vi "Online_Program_redesign_For_TV_1세부.vi"() -> ()   [LabVIEW 2014]
uses:
  <vilib>/Utility/file.llb/Read From Spreadsheet File (DBL).vi
  <vilib>/Analysis/Matrix/Numeric/Conversions/Array To Matrix - RA2.vi
  <vilib>/Instr/_visa.llb/VISA Configure Serial Port (Instr).vi
  <vilib>/DAQmx/create/channels.llb/DAQmx Create Channel (AI-Voltage-Basic).vi
  <vilib>/DAQmx/configure/timing.llb/DAQmx Timing (Sample Clock).vi
  <vilib>/DAQmx/read.llb/DAQmx Read (Analog 1D Wfm NChan NSamp).vi
  <vilib>/Analysis/Matrix/Numeric/Conversions/Array To Matrix - RA.vi
  <vilib>/Utility/file.llb/Write To Spreadsheet File (DBL).vi
  <vilib>/Utility/file.llb/Write To Spreadsheet File (I64).vi
  <vilib>/Analysis/Matrix/NI_Matrix.lvlib
  NeuroSky_Dll_Call/Debug/NeuroSky_Dll_Call.dll
  user32.dll
panel:
  out "에러 출력":errorcluster
  out "메시지 2":string
  out "큐사인":bool
  out "icon_온도":bool
  out "icon_용변":bool
  out "icon_자판":bool
  out "icon_응급":bool=TRUE
  out "icon_기계":bool
  out "icon_침대":bool
  out "메시지":string
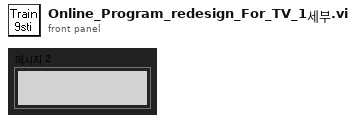
[diagram p1: front panel]
types:
  T1 = typedef "NI_Matrix.lvlib/RealMatrix.ctl" = dbl[][]
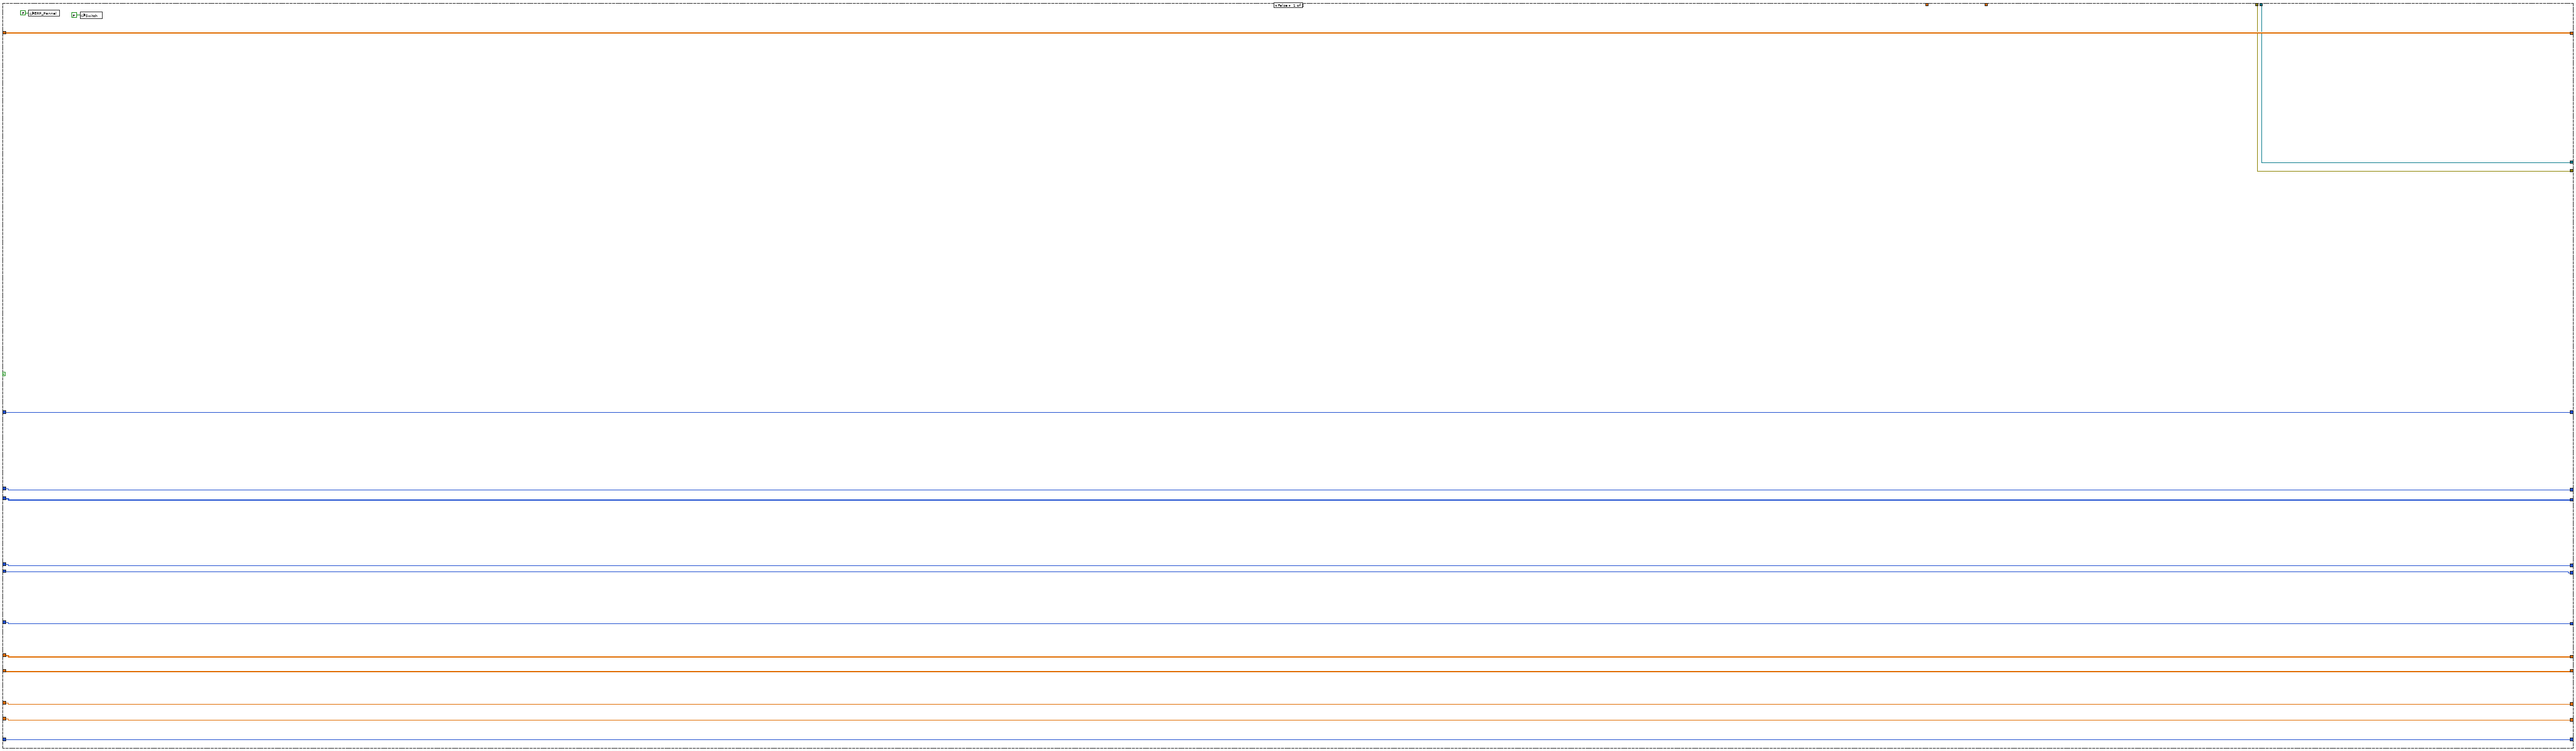
[diagram p2: hidden frame]
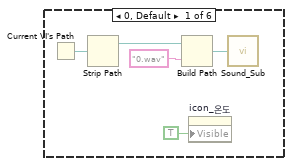
[diagram p3: hidden frame]
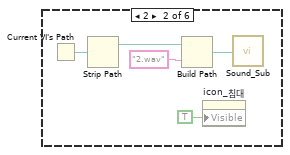
[diagram p4: hidden frame]
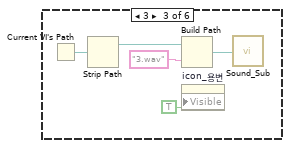
[diagram p5: hidden frame]
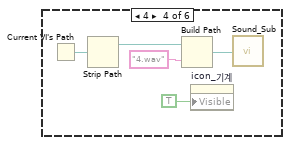
[diagram p6: hidden frame]
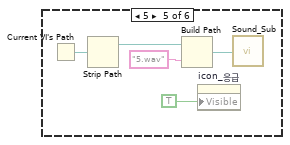
[diagram p7: hidden frame]
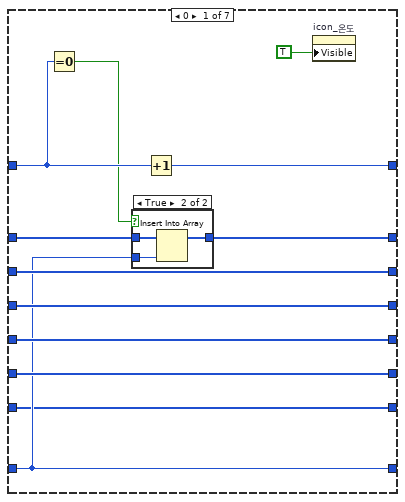
[diagram p9: hidden frame]
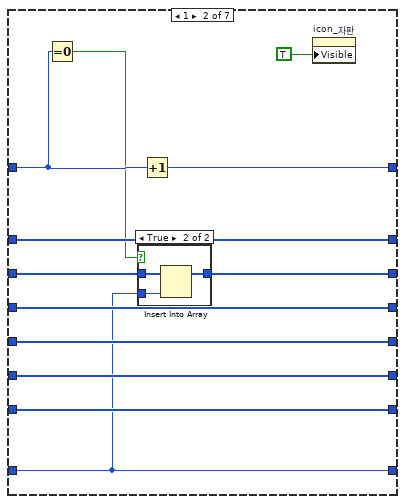
[diagram p11: hidden frame]
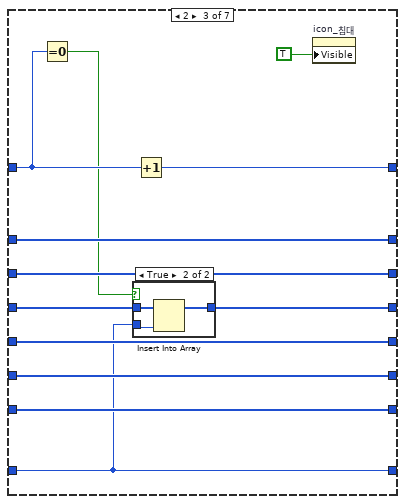
[diagram p13: hidden frame]
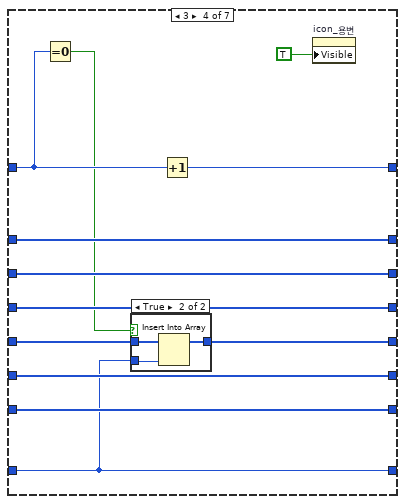
[diagram p15: hidden frame]
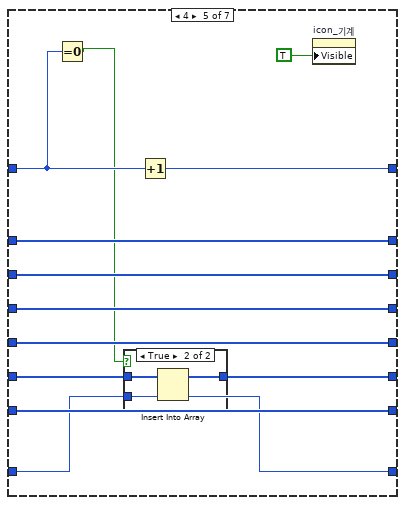
[diagram p17: hidden frame]
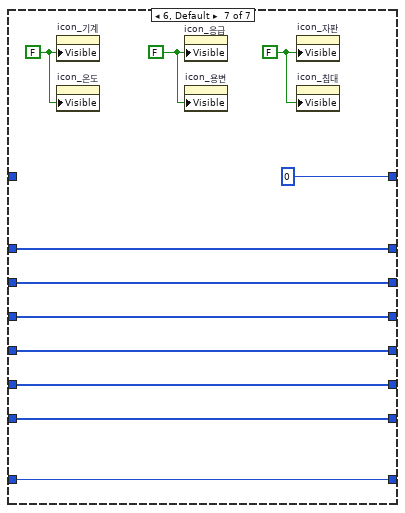
[diagram p20: hidden frame]
diagram:
  n1 = flat-sequence {
    tunnel: [w39] -> w19
    tunnel: w19 -> [w53]
    tunnel: [w53] -> w18
    tunnel: [w51] -> w17
    tunnel: [w44] -> w7
    tunnel: [w43] -> w4
    tunnel: [w40] -> w3
    tunnel: w18 -> [w72]
    tunnel: [w72] -> w16
    tunnel: [w81] -> w15
    tunnel: [w79] -> w14
    tunnel: [w77] -> w13
    tunnel: w17 -> [w61]
    tunnel: [w76] -> w12
    tunnel: [w73] -> w11
    tunnel: [w69] -> w10
    tunnel: [w67] -> w9
    tunnel: [w66] -> w8
    tunnel: w7 -> [w60]
    tunnel: [w64] -> w6
    tunnel: [w62] -> w5
    tunnel: w4 -> [w59]
    tunnel: w3 -> [w58]
    tunnel: [w57] -> w2
    tunnel: [w56] -> w1
    tunnel: w16 -> [w750]
    tunnel: w15 -> [w745]
    tunnel: w14 -> [w784]
    tunnel: w13 -> [w780]
    tunnel: w12 -> [w777]
    tunnel: w11 -> [w773]
    tunnel: w10 -> [w767]
    tunnel: w9 -> [w762]
    tunnel: w8 -> [w759]
    tunnel: w6 -> [w756]
    tunnel: w5 -> [w751]
    tunnel: w2 -> [w747]
    tunnel: w1 -> [w746]
    frame #0 {
      w20 = FALSE ("Visible")
      w22 = 500 ("Position:Left")
      # "0 = 온도\n1 = 자판\n2 = 침대\n3 = 용변 \n4 = 기계 \n5 = 응급"
      n2 = global read "Control_Panel_정리.vi" "피험자 이름"() -> (w30:string)
      n3 = Get Date/Time In Seconds() -> (seconds since 1Jan1904=w36:timestamp)
      n4 = property on="icon_기계" class="Bool (strict)"("Left"=w22, "Top"=w22) -> ()  [unwired: 2 in, 2 out]
      n5 = property on="icon_자판" class="Bool (strict)"("Left"=w22, "Top"=w22) -> ()  [unwired: 2 in, 2 out]
      n6 = property on="icon_침대" class="Bool (strict)"("Left"=w22, "Top"=w22) -> ()  [unwired: 2 in, 2 out]
      n7 = property on="icon_온도" class="Bool (strict)"("Left"=w22, "Top"=w22) -> ()  [unwired: 2 in, 2 out]
      n8 = property on="icon_용변" class="Bool (strict)"("Left"=w22, "Top"=w22) -> ()  [unwired: 2 in, 2 out]
      n9 = property on="icon_응급" class="Bool (strict)"("Left"=w22, "Top"=w22) -> ()  [unwired: 2 in, 2 out]
      n10 = property on="큐사인" class="Bool (strict)"("Left"=w22, "Top"=w22) -> ()  [unwired: 2 in, 2 out]
      n11 = Get Date/Time String(seconds (now)=w36) -> (date string=w37:string)  [unwired: 2 in, 1 out]
      n12 = Concatenate Strings("Emotion_Research\\" ("string"), w30, "_Online(Step2)\\" ("문자열")) -> (w32:string)
      n13 = Concatenate Strings(w32, w37) -> (w34:string)
      n14 = Build Path(base path=path "C:/" ("path"), name or relative path=w34) -> (appended path=w35:path)
      n15 = property on="icon_기계" class="Bool (strict)"("Visible"=w20) -> ()  [unwired: 2 in, 2 out]
      n16 = property on="icon_온도" class="Bool (strict)"("Visible"=w20) -> ()  [unwired: 2 in, 2 out]
      n17 = property on="icon_용변" class="Bool (strict)"("Visible"=w20) -> ()  [unwired: 2 in, 2 out]
      n18 = property on="icon_응급" class="Bool (strict)"("Visible"=w20) -> ()  [unwired: 2 in, 2 out]
      n19 = property on="icon_자판" class="Bool (strict)"("Visible"=w20) -> ()  [unwired: 2 in, 2 out]
      n20 = property on="icon_침대" class="Bool (strict)"("Visible"=w20) -> ()  [unwired: 2 in, 2 out]
      n21 = property on="큐사인" class="Bool (strict)"("Visible"=w20) -> ()  [unwired: 2 in, 2 out]
      n22 = Create Folder(path (use dialog)=w35) -> (created path=w39:path, error out=→"에러 출력":errorcluster)  [unwired: 2 in, 1 out]
      "icon_온도" <- FALSE ("icon_전원 6")
      "icon_용변" <- FALSE ("icon_전체종료")
      "icon_자판" <- FALSE ("icon_음량업 2")
      "icon_응급" <- FALSE ("icon_채널다운")
      "icon_기계" <- FALSE ("icon_음량다")
      "icon_침대" <- FALSE ("icon_채널업")
      "큐사인" <- FALSE ("icon_전원 7")
    }
    frame #1 {
      w47 = 1 ("인덱스 (행)")
      # "call SWLDA in matrix"
      # "call SWLDA LDA matrix"
      # "Device Control Part\ncall dll to communicate with\nNeuroSky MindWave System"
      n23 = while {
        stop <- w54 stop-if-true
        n24 = global read "Control_Panel_정리.vi" "Start"() -> (w54:bool)
      }
      n25 = global read "Control_Panel_정리.vi" "VISA resource name"() -> (w41:refnum<visa-resource-name>)
      n26 = global read "Control_Panel_정리.vi" "in"() -> (w45:path)
      n27 = global read "Control_Panel_정리.vi" "LDA_Matrix"() -> (w50:path)
      n28 = call-poly "VISA Configure Serial Port"("VISA resource name"=w41, "baud rate (9600)"=u32 115200) -> ("VISA resource name out"=w43:refnum<visa-resource-name>, "error out"=w40:errorcluster)  [unwired: 12 in]
      n29 = call-poly <vilib>:"Read From Spreadsheet File.vi"("format (%.3f)"="%.6f", "file path (dialog if empty)"=w45) -> ("all rows"=w46:dbl[][])  [unwired: 5 in, 4 out]
      n30 = call-poly <vilib>:"Read From Spreadsheet File.vi"("format (%.3f)"="%.6f", "file path (dialog if empty)"=w50) -> ("all rows"=w51:dbl[][])  [unwired: 5 in, 4 out]
      n31 = global write "Control_Panel_정리.vi" "error out"(w40) -> ()
      n32 = Delete From Array(array=w46, length=w47, index (row)=w47) -> (array with subset deleted=w48:dbl[][])  [unwired: 1 in, 1 out]
      n33 = call-poly <vilib>:"Array To Matrix.vi"("Real 2D Array"=w48) -> ("Real Matrix"=w44:T1)
    }
    frame #2 {
      w65 = dbl[] []
      w63 = dbl[][] []
      w68 = i16[] []
      n34 = while {
        shift-right: [w89] -> w81
        shift-left: dbl[][] [] -> [w95]
        shift-right: [w115] -> _
        shift-left: 0 ("y") -> [w116]
        shift-right: [w109] -> w79
        shift-left: i32[][] [] -> [w110]
        shift-right: [w113] -> w77
        shift-left: i32[] [] -> [w114]
        shift-right: [w111] -> w76
        shift-left: w68 -> [w112]
        shift-right: [w107] -> w73
        shift-left: w68 -> [w108]
        shift-right: [w106] -> w69
        shift-left: w68 -> [w105]
        shift-right: [w104] -> w67
        shift-left: w63 -> [w103]
        shift-right: [w102] -> w66
        shift-left: w65 -> [w101]
        shift-right: [w100] -> w64
        shift-left: w65 -> [w99]
        shift-right: [w98] -> w62
        shift-left: w63 -> [w97]
        tunnel: w61 -> [w96]
        tunnel: w60 -> [w94]
        tunnel: [w92] -> _
        tunnel: w59 -> [w92]
        tunnel: w58 -> [w93]
        tunnel: [w91] -> w57
        tunnel: [w90] -> w56
        shift-right: [w83] -> _
        shift-left: 0 -> [w84]
        stop <- w85 stop-if-true
        n35 = global read "Control_Panel_정리.vi" "Receive_Interaction"() -> (w87:u8)
        n36 = global read "Control_Panel_정리.vi" "Switch"() -> (w86:bool)
        n37 = dll-call lib="User32.dll" fn="GetAsyncKeyState"("vKey"=w87) -> ("return type"=w88:i64)  [unwired: 4 in, 2 out]
        n38 = Not Equal To 0?(x=w88) -> (x != 0?=w82:bool)
        n39 = Or(x=w82, y=w86) -> ()  [unwired: 1 out]
        n40 = case shown="True" w82 {
          tunnel: w116 -> [w127 w164]
          tunnel: [w127 w163] -> w115
          tunnel: w114 -> [w126 w162]
          tunnel: [w126 w161] -> w113
          tunnel: w112 -> [w123 w160]
          tunnel: [w123 w159] -> w111
          tunnel: w110 -> [w125 w158]
          tunnel: [w125 w157] -> w109
          tunnel: w108 -> [w124 w156]
          tunnel: [w124 w155] -> w107
          tunnel: [w122 w154] -> w106
          tunnel: w105 -> [w122 w153]
          tunnel: [w121 w152] -> w104
          tunnel: w103 -> [w121 w151]
          tunnel: [w119 w150] -> w102
          tunnel: w101 -> [w119 w149]
          tunnel: [w118 w148] -> w100
          tunnel: w99 -> [w118 w147]
          tunnel: [w120 w146] -> w98
          tunnel: w97 -> [w120 w145]
          tunnel: w96 -> [_ w144]
          tunnel: w95 -> [w130 w143]
          tunnel: w94 -> [_ w141]
          tunnel: w93 -> [w128 w140]
          tunnel: w92 -> [w129 w139]
          tunnel: [w129 w138] -> w91
          tunnel: [w128 w137] -> w90
          tunnel: [w130 w136] -> w89
          tunnel: w84 -> [w117 w134]
          tunnel: [w117 w133] -> w83
          frame False {
            n41 = global write "Control_Panel_정리.vi" "ERP_Pannel"(FALSE ("ERP_Pannel")) -> ()
            n42 = global write "Control_Panel_정리.vi" "Switch"(FALSE ("Switch")) -> ()
          }
          frame True {
            n43 = global write "Control_Panel_정리.vi" "ERP_Pannel"(TRUE ("ERP_Pannel")) -> ()
            n44 = flat-sequence {
              tunnel: [w216] -> w202
              tunnel: w164 -> [w215]
              tunnel: [w215] -> w201
              tunnel: [w203] -> w200
              tunnel: w162 -> [w212]
              tunnel: [w212] -> w199
              tunnel: w160 -> [w211]
              tunnel: [w211] -> w198
              tunnel: w158 -> [w210]
              tunnel: [w210] -> w197
              tunnel: [w209] -> w196
              tunnel: w156 -> [w209]
              tunnel: w153 -> [w208]
              tunnel: [w208] -> w195
              tunnel: w151 -> [w207]
              tunnel: [w207] -> w194
              tunnel: w149 -> [w206]
              tunnel: [w206] -> w193
              tunnel: w147 -> [w205]
              tunnel: [w205] -> w192
              tunnel: w145 -> [w204]
              tunnel: [w204] -> w191
              tunnel: w202 -> [w278]
              tunnel: w201 -> [w275]
              tunnel: [w276] -> w190
              tunnel: [w265] -> w189
              tunnel: [w274] -> w188
              tunnel: [w273] -> w187
              tunnel: w200 -> [w272]
              tunnel: [w272] -> w186
              tunnel: w199 -> [w271]
              tunnel: [w271] -> w185
              tunnel: [w270] -> w184
              tunnel: w198 -> [w270]
              tunnel: [w269] -> w183
              tunnel: w197 -> [w269]
              tunnel: [w268] -> w182
              tunnel: w196 -> [w268]
              tunnel: [w267] -> w181
              tunnel: w195 -> [w267]
              tunnel: [w266] -> w180
              tunnel: w194 -> [w266]
              tunnel: [w264] -> w179
              tunnel: w193 -> [w264]
              tunnel: [w263] -> w178
              tunnel: w192 -> [w263]
              tunnel: w191 -> [w262]
              tunnel: [w262] -> w177
              tunnel: w190 -> [w508]
              tunnel: w189 -> [w480]
              tunnel: w188 -> [w521]
              tunnel: w187 -> [w522]
              tunnel: w134 -> [w520]
              tunnel: [w521] -> w166
              tunnel: [w481] -> w167
              tunnel: w186 -> [w507]
              tunnel: w185 -> [w516]
              tunnel: [w515] -> w168
              tunnel: w184 -> [w513]
              tunnel: [w512] -> w169
              tunnel: w183 -> [w511]
              tunnel: [w509] -> w170
              tunnel: w182 -> [w506]
              tunnel: [w505] -> w171
              tunnel: [w503] -> w172
              tunnel: w181 -> [w502]
              tunnel: [w500] -> w173
              tunnel: w180 -> [w499]
              tunnel: [w497] -> w174
              tunnel: w179 -> [w496]
              tunnel: [w494] -> w175
              tunnel: w178 -> [w493]
              tunnel: [w490] -> w176
              tunnel: w177 -> [w489]
              tunnel: w144 -> [w488]
              tunnel: [w480] -> w142
              tunnel: w141 -> [w484]
              tunnel: [w483] -> w165
              tunnel: [w543] -> w163
              tunnel: [w542] -> w161
              tunnel: [w539] -> w159
              tunnel: [w541] -> w157
              tunnel: [w540] -> w155
              tunnel: [w538] -> w154
              tunnel: [w537] -> w152
              tunnel: [w536] -> w150
              tunnel: [w535] -> w148
              tunnel: [w534] -> w146
              tunnel: w176 -> [w534]
              tunnel: w175 -> [w535]
              tunnel: w174 -> [w536]
              tunnel: w173 -> [w537]
              tunnel: w172 -> [w538]
              tunnel: w171 -> [w540]
              tunnel: w170 -> [w541]
              tunnel: w169 -> [w539]
              tunnel: w168 -> [w542]
              tunnel: w167 -> [w533]
              tunnel: w166 -> [w543]
              tunnel: w165 -> [w532]
              tunnel: w140 -> [w531]
              tunnel: w139 -> [w530]
              tunnel: [w529] -> w138
              tunnel: [w528] -> w137
              frame #0 {
                # "결과로 만들어지는 배열은 일차원배열로\n출력되면 랜덤 숫자는 0부터 시작함"
                n45 = global read "Control_Panel_정리.vi" "Target_Command"() -> (w203:i32)
                n46 = global read "Control_Panel_정리.vi" "Flash_Repeat"() -> (w214:i32)
                n47 = global read "Control_Panel_정리.vi" "Random_num"() -> (w213:i32)
                n48 = disable-structure shown="비활성화" {
                  disable-tunnel: w203 -> [w217 _]
                  frame Disabled {
                    n49 = case shown="1" w217 {
                      frame 0, Default {
                        n50 = Current VI's Path() -> (path=w220:path)
                        n51 = Strip Path(path=w220) -> (stripped path=w221:path)  [unwired: 1 out]
                        n52 = Build Path(base path=w221, name or relative path="0.wav" ("이름 또는 상대 경로")) -> (appended path=w219:path)
                        n53 = property on="icon_온도" class="Bool (strict)"("Visible"=TRUE) -> ()  [unwired: 2 in, 2 out]
                        n54 = call "Sound_Sub.vi"("path"=w219) -> ()
                      }
                      frame 2 {
                        n55 = Current VI's Path() -> (path=w224:path)
                        n56 = Strip Path(path=w224) -> (stripped path=w225:path)  [unwired: 1 out]
                        n57 = Build Path(base path=w225, name or relative path="2.wav" ("이름 또는 상대 경로")) -> (appended path=w227:path)
                        n58 = property on="icon_침대" class="Bool (strict)"("Visible"=TRUE) -> ()  [unwired: 2 in, 2 out]
                        n59 = call "Sound_Sub.vi"("path"=w227) -> ()
                      }
                      frame 3 {
                        n60 = Current VI's Path() -> (path=w229:path)
                        n61 = Strip Path(path=w229) -> (stripped path=w230:path)  [unwired: 1 out]
                        n62 = Build Path(base path=w230, name or relative path="3.wav" ("이름 또는 상대 경로")) -> (appended path=w232:path)
                        n63 = property on="icon_용변" class="Bool (strict)"("Visible"=TRUE) -> ()  [unwired: 2 in, 2 out]
                        n64 = call "Sound_Sub.vi"("path"=w232) -> ()
                      }
                      frame 4 {
                        n65 = Current VI's Path() -> (path=w234:path)
                        n66 = Strip Path(path=w234) -> (stripped path=w235:path)  [unwired: 1 out]
                        n67 = Build Path(base path=w235, name or relative path="4.wav" ("이름 또는 상대 경로")) -> (appended path=w237:path)
                        n68 = property on="icon_기계" class="Bool (strict)"("Visible"=TRUE) -> ()  [unwired: 2 in, 2 out]
                        n69 = call "Sound_Sub.vi"("path"=w237) -> ()
                      }
                      frame 5 {
                        n70 = Current VI's Path() -> (path=w239:path)
                        n71 = Strip Path(path=w239) -> (stripped path=w240:path)  [unwired: 1 out]
                        n72 = Build Path(base path=w240, name or relative path="5.wav" ("이름 또는 상대 경로")) -> (appended path=w242:path)
                        n73 = property on="icon_응급" class="Bool (strict)"("Visible"=TRUE) -> ()  [unwired: 2 in, 2 out]
                        n74 = call "Sound_Sub.vi"("path"=w242) -> ()
                      }
                      frame 1 {
                        n75 = Current VI's Path() -> (path=w245:path)
                        n76 = Strip Path(path=w245) -> (stripped path=w246:path)  [unwired: 1 out]
                        n77 = Build Path(base path=w246, name or relative path="1.wav" ("이름 또는 상대 경로")) -> (appended path=w244:path)
                        n78 = property on="icon_자판" class="Bool (strict)"("Visible"=TRUE) -> ()  [unwired: 2 in, 2 out]
                        n79 = call "Sound_Sub.vi"("path"=w244) -> ()
                      }
                    }
                  }
                  frame Enabled {
                  }
                }
                n80 = call "Random2.vi"("Random_num"=w213, "전체횟수"=w214) -> ("배열"=w216:i32[])
              }
              frame #1 {
                n81 = flat-sequence {
                  tunnel: w275 -> [w280]
                  tunnel: w278 -> [w281]
                  tunnel: [w281] -> w261
                  tunnel: [w280] -> w260
                  tunnel: [w284] -> w253
                  tunnel: [w283] -> w252
                  tunnel: w261 -> [w284]
                  tunnel: w260 -> [w283]
                  tunnel: w253 -> [w287]
                  tunnel: [w287] -> w251
                  tunnel: w252 -> [w286]
                  tunnel: [w286] -> w249
                  tunnel: w251 -> [w290]
                  tunnel: [w290] -> w250
                  tunnel: w249 -> [w289]
                  tunnel: [w289] -> w248
                  tunnel: w250 -> [w326]
                  tunnel: w248 -> [w316]
                  tunnel: [w324] -> w254
                  tunnel: [w323] -> w255
                  tunnel: [w322] -> w257
                  tunnel: [w321] -> w258
                  tunnel: [w320] -> w259
                  tunnel: [w315] -> w274
                  tunnel: [w314] -> w273
                  tunnel: [w313] -> w256
                  tunnel: [w312] -> w265
                  frame #0 {
                    w279 = FALSE ("Visible")
                    # "모든 자극을 시작전에\n꺼줌"
                    n82 = property on="icon_기계" class="Bool (strict)"("Visible"=w279) -> ()  [unwired: 2 in, 2 out]
                    n83 = property on="icon_온도" class="Bool (strict)"("Visible"=w279) -> ()  [unwired: 2 in, 2 out]
                    n84 = property on="icon_용변" class="Bool (strict)"("Visible"=w279) -> ()  [unwired: 2 in, 2 out]
                    n85 = property on="icon_응급" class="Bool (strict)"("Visible"=w279) -> ()  [unwired: 2 in, 2 out]
                    n86 = property on="icon_자판" class="Bool (strict)"("Visible"=w279) -> ()  [unwired: 2 in, 2 out]
                    n87 = property on="icon_침대" class="Bool (strict)"("Visible"=w279) -> ()  [unwired: 2 in, 2 out]
                  }
                  frame #1 {
                    n88 = property on="큐사인" class="Bool (strict)"("Visible"=TRUE) -> ()  [unwired: 2 in, 2 out]
                  }
                  frame #2 {
                    # "2초간 큐사인 유지"
                    n89 = Wait (ms)(milliseconds to wait=u32 2000) -> ()  [unwired: 1 out]
                  }
                  frame #3 {
                    # "자극 제시와 동시에 cue사인은\n사라짐"
                    n90 = property on="큐사인" class="Bool (strict)"("Visible"=FALSE) -> ()  [unwired: 2 in, 2 out]
                  }
                  frame #4 {
                    w318 = i32[] []
                    # "이 프로그램 실행시\nRate = 512Hz\nFrame Length = 40\n으로 세팅하여서 시작하여아함"
                    # "마지막 자극제시 후\n1초데이터를 받기 위해 2초에\n해당하는 frame 수만큼 반복\n횟수를 추가함"
                    n91 = global read "Control_Panel_정리.vi" "Frame Length"() -> (w296:i32)
                    n92 = global read "Control_Panel_정리.vi" "sample mode"() -> (w298:i32)
                    n93 = global read "Control_Panel_정리.vi" "input terminal configuration"() -> (w300:i32)
                    n94 = global read "Control_Panel_정리.vi" "rate"() -> (w297:dbl)
                    n95 = global read "Control_Panel_정리.vi" "physical channels"() -> (w299:tag)
                    n96 = call-poly <vilib>:"DAQmx Create Virtual Channel.vi"("maximum value"=10.0, "minimum value"=-10.0, "input terminal configuration"=w300, "physical channels"=w299) -> ("task out"=w304:refnum<k21>, "error out"=w307:errorcluster)  [unwired: 10 in]
                    n97 = call-poly <vilib>:"DAQmx Timing.vi"("task/channels in"=w304, "sample mode"=w298, "samples per channel"=w296, "rate"=w297, "error in"=w307) -> ("task out"=w303:refnum<k21>, "error out"=w308:errorcluster)  [unwired: 9 in]
                    n98 = global read "Control_Panel_정리.vi" "rate"() -> (w310:dbl)
                    n99 = global read "Control_Panel_정리.vi" "Frame Length"() -> (w309:i32)
                    n100 = call <vilib>:"DAQmx Start Task.vi"("task/channels in"=w303, "error in"=w308) -> ("task out"=w305:refnum<k21>, "error out"=w306:errorcluster)  [unwired: 12 in]
                    n101 = Divide(x=w310, y=w309) -> (x/y=w311:dbl)
                    n102 = while {
                      tunnel: w326 -> [w370]
                      shift-right: [w329] -> w312
                      shift-left: dbl[][] [] -> [w331]
                      shift-right: [w367] -> w324
                      shift-left: w318 -> [w366]
                      shift-right: [w364] -> w323
                      shift-left: w318 -> [w365]
                      shift-right: [w362] -> w313
                      shift-left: w318 -> [w363]
                      shift-right: [w360] -> w322
                      shift-left: w318 -> [w361]
                      shift-right: [w358] -> w321
                      shift-left: w318 -> [w359]
                      shift-right: [w357] -> w320
                      shift-left: w318 -> [w344]
                      shift-right: [w355] -> w315
                      shift-left: w316 -> [w356]
                      shift-right: [w351] -> _
                      shift-left: 0 -> [w350]
                      shift-right: [w345] -> _
                      shift-left: 0 ("y") -> [w346]
                      tunnel: [w340] -> w314
                      tunnel: w311 -> [w336]
                      tunnel: w306 -> [w333]
                      tunnel: w305 -> [w334]
                      tunnel: w296 -> [w332]
                      tunnel: [w328] -> w292
                      tunnel: [w327] -> w291
                      i -> [w340]
                      stop <- w371 stop-if-true
                      # "ITR  = 240ms + 40ms = 280ms"
                      # "현재 stimulus가 시작된 이후\n1) 현재까지 받은 frame 수가 6개 이하면\n계속 현재 stimulus를 켜 놓는다\n2) 현재 받는 frame이 7번째 이면\nstimulus를 1개 프레임 시간 (40ms)동안\n끈고 다음 stimulus로 넘어간다."
                      # "Stimulus 순서에 따른 아이콘\n\n\n0 = 온도\n1 = 자판\n2 = 침대\n3 = 용변 \n4 = 기계 \n5 = 응급"
                      # "Stimulus 5"
                      # "Stimulus 4"
                      # "Stimulus 3"
                      # "Stimulus 2"
                      # "Stimulus 1"
                      # "Stimulus 0"
                      n103 = call-poly <vilib>:"DAQmx Read.vi"("task/channels in"=w334, "number of samples per channel"=w332, "error in"=w333) -> ("task out"=w328:refnum<k21>, "data"=w335:waveform(dbl)[], "error out"=w327:errorcluster)  [unwired: 10 in]
                      n104 = call "다이나믹 데이터로부터 변환"("Dynamic Data Type"=w335) -> ("Array"=w330:dbl[][])  [unwired: 3 in]
                      n105 = Build Array (concatenate)(w331, w330) -> (w329:dbl[][])
                      n106 = global read "Control_Panel_정리.vi" "Random_num"() -> (w339:i32)
                      n107 = global read "Control_Panel_정리.vi" "Flash_Repeat"() -> (w338:i32)
                      n108 = Round Toward -Infinity(1:w336) -> (0:w337:dbl)
                      n109 = Increment(x=w340) -> (x+1=w343:i32)
                      n110 = Multiply(x=w339, y=w338) -> (x*y=w341:i32)
                      n111 = Quotient & Remainder(x=w343, y=3) -> (x-y*floor(x/y)=w353:i32)  [unwired: 1 out]
                      n112 = Add(x=w337, y=w341) -> (x+y=w372:dbl)
                      n113 = Equal To 0?(x=w353) -> (x = 0?=w349:bool)
                      n114 = Greater Or Equal?(x=w350, y=w372) -> (x >= y?=w371:bool)
                      n115 = Greater Or Equal?(x=w350, y=w341) -> (x >= y?=w348:bool)
                      n116 = Increment(x=w356) -> (x+1=w368:i32)
                      n117 = Index Array(array=w370, index=w350) -> (element=w342:i32)
                      n118 = Or(x=w349, y=w348) -> (x .or. y?=w347:bool)
                      n119 = Increment(x=w350) -> (x+1=w352:i32)
                      n120 = Select(t=w352, s=w349, f=w350) -> (s? t:f=w351:i32)
                      n121 = Select(t=w339, s=w347, f=w342) -> (s? t:f=w369:i32)
                      n122 = case shown="5" w369 {
                        tunnel: w368 -> [w378 w394 w409 w425 w441 w458 w473]
                        tunnel: [w383 w391 w416 w432 w448 w464 w479] -> w367
                        tunnel: w366 -> [w384 w391 w416 w432 w448 w464 w479]
                        tunnel: w365 -> [w382 w400 w413 w429 w445 w462 w478]
                        tunnel: [w382 w399 w413 w429 w445 w462 w478] -> w364
                        tunnel: w363 -> [w381 w398 w415 w428 w444 w461 w477]
                        tunnel: [w381 w398 w414 w428 w444 w461 w477] -> w362
                        tunnel: w361 -> [w380 w397 w412 w431 w443 w460 w476]
                        tunnel: [w380 w397 w412 w430 w443 w460 w476] -> w360
                        tunnel: w359 -> [w379 w396 w411 w427 w447 w459 w475]
                        tunnel: [w379 w396 w411 w427 w446 w459 w475] -> w358
                        tunnel: w344 -> [w375 w395 w410 w426 w442 w463 w474]
                        tunnel: [w375 w395 w410 w426 w442 w455 w474] -> w357
                        tunnel: [w378 w394 w409 w425 w441 w458 w473] -> w355
                        tunnel: w346 -> [w377 w393 w408 w423 w440 w456 _]
                        tunnel: [w376 w392 w407 w424 w439 w457 0] -> w345
                        frame 0 {
                          n123 = Equal To 0?(x=w377) -> (x = 0?=w373:bool)
                          n124 = case shown="True" w373 {
                            tunnel: w384 -> [w385 w388]
                            tunnel: [w385 w387] -> w383
                            tunnel: w378 -> [_ w386]
                            frame False {
                            }
                            frame True {
                              n125 = Insert Into Array(array=w388, new element=w386) -> (w387:i32[])  [unwired: 1 in]
                            }
                          }
                          n126 = Increment(x=w377) -> (x+1=w376:i32)
                          n127 = property on="icon_온도" class="Bool (strict)"("Visible"=TRUE) -> ()  [unwired: 2 in, 2 out]
                        }
                        frame 1 {
                          n128 = Equal To 0?(x=w393) -> (x = 0?=w389:bool)
                          n129 = case shown="True" w389 {
                            tunnel: w400 -> [w401 w404]
                            tunnel: [w401 w403] -> w399
                            tunnel: w394 -> [_ w402]
                            frame False {
                            }
                            frame True {
                              n130 = Insert Into Array(array=w404, new element=w402) -> (w403:i32[])  [unwired: 1 in]
                            }
                          }
                          n131 = Increment(x=w393) -> (x+1=w392:i32)
                          n132 = property on="icon_자판" class="Bool (strict)"("Visible"=TRUE) -> ()  [unwired: 2 in, 2 out]
                        }
                        frame 2 {
                          n133 = Equal To 0?(x=w408) -> (x = 0?=w405:bool)
                          n134 = case shown="True" w405 {
                            tunnel: w415 -> [w417 w420]
                            tunnel: [w417 w419] -> w414
                            tunnel: w409 -> [_ w418]
                            frame False {
                            }
                            frame True {
                              n135 = Insert Into Array(array=w420, new element=w418) -> (w419:i32[])  [unwired: 1 in]
                            }
                          }
                          n136 = Increment(x=w408) -> (x+1=w407:i32)
                          n137 = property on="icon_침대" class="Bool (strict)"("Visible"=TRUE) -> ()  [unwired: 2 in, 2 out]
                        }
                        frame 3 {
                          n138 = Equal To 0?(x=w423) -> (x = 0?=w421:bool)
                          n139 = case shown="True" w421 {
                            tunnel: w431 -> [w433 w436]
                            tunnel: [w433 w435] -> w430
                            tunnel: w425 -> [_ w434]
                            frame False {
                            }
                            frame True {
                              n140 = Insert Into Array(array=w436, new element=w434) -> (w435:i32[])  [unwired: 1 in]
                            }
                          }
                          n141 = Increment(x=w423) -> (x+1=w424:i32)
                          n142 = property on="icon_용변" class="Bool (strict)"("Visible"=TRUE) -> ()  [unwired: 2 in, 2 out]
                        }
                        frame 4 {
                          n143 = Equal To 0?(x=w440) -> (x = 0?=w437:bool)
                          n144 = case shown="True" w437 {
                            tunnel: w447 -> [w449 w452]
                            tunnel: [w449 w451] -> w446
                            tunnel: w441 -> [_ w450]
                            frame False {
                            }
                            frame True {
                              n145 = Insert Into Array(array=w452, new element=w450) -> (w451:i32[])  [unwired: 1 in]
                            }
                          }
                          n146 = Increment(x=w440) -> (x+1=w439:i32)
                          n147 = property on="icon_기계" class="Bool (strict)"("Visible"=TRUE) -> ()  [unwired: 2 in, 2 out]
                        }
                        frame 5 {
                          n148 = Equal To 0?(x=w456) -> (x = 0?=w453:bool)
                          n149 = case shown="True" w453 {
                            tunnel: w463 -> [w465 w468]
                            tunnel: [w465 w467] -> w455
                            tunnel: w458 -> [_ w466]
                            frame False {
                            }
                            frame True {
                              n150 = Insert Into Array(array=w468, new element=w466) -> (w467:i32[])  [unwired: 1 in]
                            }
                          }
                          n151 = Increment(x=w456) -> (x+1=w457:i32)
                          n152 = property on="icon_응급" class="Bool (strict)"("Visible"=TRUE) -> ()  [unwired: 2 in, 2 out]
                        }
                        frame 6, Default {
                          w470 = FALSE ("Visible")
                          w471 = FALSE ("Visible")
                          w469 = FALSE ("Visible")
                          n153 = property on="icon_기계" class="Bool (strict)"("Visible"=w469) -> ()  [unwired: 2 in, 2 out]
                          n154 = property on="icon_온도" class="Bool (strict)"("Visible"=w469) -> ()  [unwired: 2 in, 2 out]
                          n155 = property on="icon_응급" class="Bool (strict)"("Visible"=w471) -> ()  [unwired: 2 in, 2 out]
                          n156 = property on="icon_용변" class="Bool (strict)"("Visible"=w471) -> ()  [unwired: 2 in, 2 out]
                          n157 = property on="icon_자판" class="Bool (strict)"("Visible"=w470) -> ()  [unwired: 2 in, 2 out]
                          n158 = property on="icon_침대" class="Bool (strict)"("Visible"=w470) -> ()  [unwired: 2 in, 2 out]
                        }
                      }
                    }
                    n159 = call <vilib>:"DAQmx Stop Task.vi"("task/channels in"=w292, "error in"=w291) -> ("task out"=w293:refnum<k21>, "error out"=w294:errorcluster)  [unwired: 12 in]
                    n160 = call <vilib>:"DAQmx Clear Task.vi"("task in"=w293, "error in"=w294) -> ("error out"=w295:errorcluster)  [unwired: 13 in]
                    n161 = call <vilib>:"Simple Error Handler.vi"("error in (no error)"=w295) -> ()  [unwired: 4 in, 5 out]
                  }
                }
                n162 = Build Array(w254, w255, w256, w257, w258, w259) -> (w277:i32[][])
                n163 = Transpose 2D Array(2D array=w277) -> (transposed array=w276:i32[][])
              }
              frame #2 {
                w525 = 1 ("인덱스 (행)")
                # "각 stimulus 구간에서 EEG\n(ERP_total.txt라 저장됨)"
                # "ERP parameter값"
                # "SVM의 decision 값"
                # "SWLDA_hyperplane 값"
                # "ERP_발생_Total\n(ERP 발생 여부)"
                # "Target Order"
                # "Flash order"
                # "이 열의 행렬들 \n(위에서 아래로)\n1) Stimulus order array\n2) Accuracy array"
                n164 = Increment(x=w522) -> (x+1=w526:i32)
                n165 = Multiply(x=w526, y=w520) -> (x*y=w527:i32)
                n166 = Subtract(x=w508, y=w527) -> (x-y=w510:i32[][])
                n167 = Delete From Array(array=w488, length=w525, index (row)=w525) -> (array with subset deleted=w486:dbl[][])  [unwired: 1 in, 1 out]
                n168 = global read "Control_Panel_정리.vi" "rate"() -> (w518:dbl)
                n169 = global read "Control_Panel_정리.vi" "Frame Length"() -> (w519:i32)
                n170 = call-poly <vilib>:"Array To Matrix.vi"("Real 2D Array"=w486) -> ("Real Matrix"=w485:T1)
                n171 = Index Array(array=w486, index (col)=0 ("인덱스")) -> (element=w487:dbl[])  [unwired: 1 in]
                n172 = call-poly <vilib>:"Array To Matrix.vi"("Real 1D Array"=w487) -> ("Real Matrix (Column Vector)"=w523:T1)
                n173 = call "Subvi_Online_SVM_SWLDA_1세부통합.vi"("rate"=w518, "Value"=w523, "Matrix"=w485, "in"=w484, "samples per channel"=w519, "Brain_data_source"=w480, "Target_Flash_Order"=w510) -> ("output-0~8"=w481:i32, "decision"=w495:dbl[], "ERP_발생여부"=w483:bool, "SWLDA"=w498:dbl[], "EPR_발생_total"=w504:i16[], "ERP_all"=w492:dbl[][], "ERP_Parameters"=w501:dbl[][])  [unwired: 2 in]
                n174 = Transpose 2D Array(2D array=w492) -> (transposed array=w491:dbl[][])
                n175 = Build Array (concatenate)(w502, w504) -> (w503:i16[])
                n176 = Build Array (concatenate)(w499, w501) -> (w500:dbl[][])
                n177 = Build Array (concatenate)(w489, w491) -> (w490:dbl[][])
                n178 = Build Array (concatenate)(w496, w498) -> (w497:dbl[])
                n179 = Build Array (concatenate)(w493, w495) -> (w494:dbl[])
                n180 = Build Array (concatenate)(w506, w507) -> (w505:i32[])
                n181 = Build Array (concatenate)(w511, w510) -> (w509:i32[][])
                n182 = global read "Control_Panel_정리.vi" "Target_Command"() -> (w482:i32)
                n183 = Equal?(x=w481, y=w507) -> (x = y?=w517:bool)
                n184 = Boolean To (0,1)(Boolean=w517) -> (0, 1=w514:i16)
                n185 = Build Array (concatenate)(w516, w481) -> (w515:i32[])
                n186 = Build Array (concatenate)(w513, w514) -> (w512:i16[])
                n187 = Equal?(x=w482, y=w481) -> ()  [unwired: 1 out]
              }
              frame #3 {
                # "0 = 온도\n1 = 자판\n2 = 침대\n3 = 용변 \n4 = 기계 \n5 = 응급"
                n188 = disable-structure shown="활성화" {
                  disable-tunnel: w533 -> [w551 w706]
                  disable-tunnel: w532 -> [w550 w705]
                  disable-tunnel: w531 -> [w549 _]
                  disable-tunnel: w530 -> [w548 _]
                  disable-tunnel: [w547 _] -> w529
                  disable-tunnel: [w546 _] -> w528
                  frame Enabled {
                    n189 = flat-sequence {
                      tunnel: w551 -> [w558]
                      tunnel: w550 -> [_]
                      tunnel: w549 -> [w557]
                      tunnel: w548 -> [w556]
                      tunnel: [w555] -> w545
                      tunnel: [w554] -> w544
                      tunnel: [w695] -> w546
                      tunnel: [w696] -> w547
                      tunnel: w545 -> [w696]
                      tunnel: w544 -> [w695]
                      frame #0 {
                        n190 = case shown="True" TRUE {
                          tunnel: w558 -> [_ w567]
                          tunnel: ["No Decesion" ("메시지") w566] -> w553
                          tunnel: w557 -> [w559 w565]
                          tunnel: w556 -> [w560 w564]
                          tunnel: [w560 w563] -> w555
                          tunnel: [w559 w562] -> w554
                          frame False {
                          }
                          frame True {
                            n191 = disable-structure shown="Enabled" {
                              disable-tunnel: [w573 _ "" ("메시지")] -> w566
                              disable-tunnel: w567 -> [w568 w667 _]
                              disable-tunnel: w565 -> [w572 _ _]
                              disable-tunnel: w564 -> [w571 _ _]
                              disable-tunnel: [w570 _ _] -> w563
                              disable-tunnel: [w569 _ _] -> w562
                              frame Enabled {
                                n192 = case shown="3" w568 {
                                tunnel: ["전원" ("메시지") "음향 UP" ("메시지") "채널 UP" ("메시지") "전체종료" ("메시지") "음향 Down" ("메시지") "채널 Down" ("메시지") "No Decesion" ("메시지")] -> w573
                                tunnel: w572 -> [w579 w594 w609 w621 w639 w654 w664]
                                tunnel: w571 -> [w575 w590 w605 w622 w635 w650 w665]
                                tunnel: [w578 w593 w608 w620 w638 w653 w665] -> w570
                                tunnel: [w577 w592 w607 w619 w637 w652 w664] -> w569
                                frame 0 {
                                n193 = flat-sequence {
                                tunnel: w579 -> [w583]
                                tunnel: [w583] -> w576
                                tunnel: w575 -> [w582]
                                tunnel: [w582] -> w574
                                tunnel: [w586] -> w578
                                tunnel: [w585] -> w577
                                tunnel: w576 -> [w587]
                                tunnel: w574 -> [w584]
                                frame #0 {
                                n194 = Wait (ms)(milliseconds to wait=u32 100) -> ()  [unwired: 1 out]
                                }
                                frame #1 {
                                n195 = VISA Write(VISA resource name=w584, write buffer="0", error in (no error)=w587) -> (VISA resource name out=w586:refnum<visa-resource-name>, error out=w585:errorcluster)  [unwired: 1 out]
                                }
                                }
                                }
                                frame 1 {
                                n196 = flat-sequence {
                                tunnel: w594 -> [w598]
                                tunnel: [w598] -> w591
                                tunnel: w590 -> [w597]
                                tunnel: [w597] -> w589
                                tunnel: [w601] -> w593
                                tunnel: [w600] -> w592
                                tunnel: w591 -> [w602]
                                tunnel: w589 -> [w599]
                                frame #0 {
                                n197 = Wait (ms)(milliseconds to wait=u32 100) -> ()  [unwired: 1 out]
                                }
                                frame #1 {
                                n198 = VISA Write(VISA resource name=w599, write buffer="L", error in (no error)=w602) -> (VISA resource name out=w601:refnum<visa-resource-name>, error out=w600:errorcluster)  [unwired: 1 out]
                                }
                                }
                                }
                                frame 2 {
                                n199 = flat-sequence {
                                tunnel: w609 -> [w613]
                                tunnel: [w613] -> w606
                                tunnel: [w612] -> _
                                tunnel: w605 -> [w612]
                                tunnel: [w612] -> w604
                                tunnel: [w616] -> w608
                                tunnel: [w615] -> w607
                                tunnel: w606 -> [w617]
                                tunnel: w604 -> [w614]
                                frame #0 {
                                n200 = Wait (ms)(milliseconds to wait=u32 100) -> ()  [unwired: 1 out]
                                }
                                frame #1 {
                                n201 = VISA Write(VISA resource name=w614, write buffer="J", error in (no error)=w617) -> (VISA resource name out=w616:refnum<visa-resource-name>, error out=w615:errorcluster)  [unwired: 1 out]
                                }
                                }
                                }
                                frame 3 {
                                n202 = flat-sequence {
                                tunnel: w621 -> [w628]
                                tunnel: [w628] -> w624
                                tunnel: w622 -> [w627]
                                tunnel: [w627] -> w623
                                tunnel: [w631] -> w620
                                tunnel: [w630] -> w619
                                tunnel: w624 -> [w632]
                                tunnel: w623 -> [w629]
                                frame #0 {
                                n203 = Wait (ms)(milliseconds to wait=u32 100) -> ()  [unwired: 1 out]
                                }
                                frame #1 {
                                n204 = VISA Write(VISA resource name=w629, write buffer="0", error in (no error)=w632) -> (VISA resource name out=w631:refnum<visa-resource-name>, error out=w630:errorcluster)  [unwired: 1 out]
                                }
                                }
                                }
                                frame 4 {
                                n205 = flat-sequence {
                                tunnel: w639 -> [w643]
                                tunnel: [w643] -> w636
                                tunnel: w635 -> [w641]
                                tunnel: [w641] -> w634
                                tunnel: [w646] -> w638
                                tunnel: [w645] -> w637
                                tunnel: w636 -> [w647]
                                tunnel: w634 -> [w644]
                                frame #0 {
                                n206 = Wait (ms)(milliseconds to wait=u32 100) -> ()  [unwired: 1 out]
                                }
                                frame #1 {
                                n207 = VISA Write(VISA resource name=w644, write buffer="M", error in (no error)=w647) -> (VISA resource name out=w646:refnum<visa-resource-name>, error out=w645:errorcluster)  [unwired: 1 out]
                                }
                                }
                                }
                                frame 5 {
                                n208 = flat-sequence {
                                tunnel: w654 -> [w658]
                                tunnel: [w658] -> w651
                                tunnel: w650 -> [w657]
                                tunnel: [w657] -> w649
                                tunnel: [w661] -> w653
                                tunnel: [w660] -> w652
                                tunnel: w651 -> [w662]
                                tunnel: w649 -> [w659]
                                frame #0 {
                                n209 = Wait (ms)(milliseconds to wait=u32 100) -> ()  [unwired: 1 out]
                                }
                                frame #1 {
                                n210 = VISA Write(VISA resource name=w659, write buffer="K", error in (no error)=w662) -> (VISA resource name out=w661:refnum<visa-resource-name>, error out=w660:errorcluster)  [unwired: 1 out]
                                }
                                }
                                }
                                frame 9, Default {
                                }
                                }
                              }
                              frame Disabled {
                                n211 = case shown="0, Default" w667 {
                                frame 0, Default {
                                n212 = Current VI's Path() -> (path=w669:path)
                                n213 = Strip Path(path=w669) -> (stripped path=w670:path)  [unwired: 1 out]
                                n214 = Build Path(base path=w670, name or relative path="0.wav" ("이름 또는 상대 경로")) -> (appended path=w668:path)
                                n215 = call "Sound_Sub.vi"("path"=w668) -> ()
                                }
                                frame 2 {
                                n216 = Current VI's Path() -> (path=w672:path)
                                n217 = Strip Path(path=w672) -> (stripped path=w673:path)  [unwired: 1 out]
                                n218 = Build Path(base path=w673, name or relative path="2.wav" ("이름 또는 상대 경로")) -> (appended path=w675:path)
                                n219 = call "Sound_Sub.vi"("path"=w675) -> ()
                                }
                                frame 3 {
                                n220 = Current VI's Path() -> (path=w676:path)
                                n221 = Strip Path(path=w676) -> (stripped path=w677:path)  [unwired: 1 out]
                                n222 = Build Path(base path=w677, name or relative path="3.wav" ("이름 또는 상대 경로")) -> (appended path=w679:path)
                                n223 = call "Sound_Sub.vi"("path"=w679) -> ()
                                }
                                frame 4 {
                                n224 = Current VI's Path() -> (path=w680:path)
                                n225 = Strip Path(path=w680) -> (stripped path=w681:path)  [unwired: 1 out]
                                n226 = Build Path(base path=w681, name or relative path="4.wav" ("이름 또는 상대 경로")) -> (appended path=w683:path)
                                n227 = call "Sound_Sub.vi"("path"=w683) -> ()
                                }
                                frame 5 {
                                n228 = Current VI's Path() -> (path=w684:path)
                                n229 = Strip Path(path=w684) -> (stripped path=w685:path)  [unwired: 1 out]
                                n230 = Build Path(base path=w685, name or relative path="5.wav" ("이름 또는 상대 경로")) -> (appended path=w687:path)
                                n231 = call "Sound_Sub.vi"("path"=w687) -> ()
                                }
                                frame 1 {
                                n232 = Current VI's Path() -> (path=w689:path)
                                n233 = Strip Path(path=w689) -> (stripped path=w690:path)  [unwired: 1 out]
                                n234 = Build Path(base path=w690, name or relative path="1.wav" ("이름 또는 상대 경로")) -> (appended path=w688:path)
                                n235 = call "Sound_Sub.vi"("path"=w688) -> ()
                                }
                                }
                              }
                              frame Disabled {
                              }
                            }
                          }
                        }
                        n236 = global write "Control_Panel_정리.vi" "선택된 기능"(w553) -> ()
                      }
                      frame #1 {
                        n237 = global read "Control_Panel_정리.vi" "Send_Interaction"() -> (w693:u8)
                        n238 = stacked-sequence {
                          tunnel: w693 -> [w698 _ w703]
                          tunnel: u32 0 ("dwFlags") -> [w697 _ w702]
                          frame #0 {
                            n239 = dll-call lib="User32.dll" fn="keybd_event"("bVk"=w698, "bScan"=w697, "dwFlags"=w697, "dwExtraInfo"=w697) -> ()  [unwired: 8 in, 2 out]
                          }
                          frame #1 {
                            n240 = global write "Control_Panel_정리.vi" "Switch"(FALSE ("Switch")) -> ()
                            n241 = Wait Until Next ms Multiple(millisecond multiple=u32 250) -> ()  [unwired: 1 out]
                          }
                          frame #2 {
                            n242 = dll-call lib="User32.dll" fn="keybd_event"("bVk"=w703, "bScan"=w702, "dwFlags"=u32 2, "dwExtraInfo"=w702) -> ()  [unwired: 8 in, 2 out]
                          }
                        }
                      }
                    }
                  }
                  frame Disabled {
                    n243 = case shown="True" w705 {
                      tunnel: w706 -> [_ w709]
                      tunnel: ["No Decesion" ("메시지") w708] -> w704
                      frame False {
                      }
                      frame True {
                        n244 = disable-structure shown="활성화" {
                          disable-tunnel: [w711 _ "" ("메시지")] -> w708
                          disable-tunnel: w709 -> [w710 w719 _]
                          frame Enabled {
                            n245 = case shown="5" w710 {
                              tunnel: ["온도" ("메시지") "자판" ("메시지") "침대" ("메시지") "용변" ("메시지") "기계" ("메시지") "응급" ("메시지") "No Decesion" ("메시지")] -> w711
                              frame 0 {
                              }
                              frame 1 {
                              }
                              frame 2 {
                              }
                              frame 3 {
                              }
                              frame 4 {
                              }
                              frame 5 {
                              }
                              frame 9, Default {
                              }
                            }
                          }
                          frame Disabled {
                            n246 = case shown="4" w719 {
                              frame 0, Default {
                                n247 = Current VI's Path() -> (path=w721:path)
                                n248 = Strip Path(path=w721) -> (stripped path=w722:path)  [unwired: 1 out]
                                n249 = Build Path(base path=w722, name or relative path="0.wav" ("이름 또는 상대 경로")) -> (appended path=w720:path)
                                n250 = call "Sound_Sub.vi"("path"=w720) -> ()
                              }
                              frame 2 {
                                n251 = Current VI's Path() -> (path=w724:path)
                                n252 = Strip Path(path=w724) -> (stripped path=w725:path)  [unwired: 1 out]
                                n253 = Build Path(base path=w725, name or relative path="2.wav" ("이름 또는 상대 경로")) -> (appended path=w727:path)
                                n254 = call "Sound_Sub.vi"("path"=w727) -> ()
                              }
                              frame 3 {
                                n255 = Current VI's Path() -> (path=w728:path)
                                n256 = Strip Path(path=w728) -> (stripped path=w729:path)  [unwired: 1 out]
                                n257 = Build Path(base path=w729, name or relative path="3.wav" ("이름 또는 상대 경로")) -> (appended path=w731:path)
                                n258 = call "Sound_Sub.vi"("path"=w731) -> ()
                              }
                              frame 4 {
                                n259 = Current VI's Path() -> (path=w732:path)
                                n260 = Strip Path(path=w732) -> (stripped path=w733:path)  [unwired: 1 out]
                                n261 = Build Path(base path=w733, name or relative path="4.wav" ("이름 또는 상대 경로")) -> (appended path=w735:path)
                                n262 = call "Sound_Sub.vi"("path"=w735) -> ()
                              }
                              frame 5 {
                                n263 = Current VI's Path() -> (path=w736:path)
                                n264 = Strip Path(path=w736) -> (stripped path=w737:path)  [unwired: 1 out]
                                n265 = Build Path(base path=w737, name or relative path="5.wav" ("이름 또는 상대 경로")) -> (appended path=w739:path)
                                n266 = call "Sound_Sub.vi"("path"=w739) -> ()
                              }
                              frame 1 {
                                n267 = Current VI's Path() -> (path=w741:path)
                                n268 = Strip Path(path=w741) -> (stripped path=w742:path)  [unwired: 1 out]
                                n269 = Build Path(base path=w742, name or relative path="1.wav" ("이름 또는 상대 경로")) -> (appended path=w740:path)
                                n270 = call "Sound_Sub.vi"("path"=w740) -> ()
                              }
                            }
                          }
                          frame Disabled {
                          }
                        }
                      }
                    }
                    n271 = global write "Control_Panel_정리.vi" "선택된 기능"(w704) -> ()
                  }
                }
              }
            }
            n272 = Increment(x=w134) -> (x+1=w133:i32)
            n273 = Build Array (concatenate)(w143, w142) -> (w136:dbl[][])
          }
        }
        n274 = global read "Control_Panel_정리.vi" "정지"() -> (w85:bool)
      }
      n275 = global write "Control_Panel_정리.vi" "Acquisition Mode"(TRUE ("Device Control Enabled")) -> ()
      n276 = global write "Control_Panel_정리.vi" "Device Control Enabled"(FALSE ("Device Control Enabled")) -> ()
    }
    frame #3 {
      n277 = VISA Close(VISA resource name=w747, error in (no error)=w746) -> ()  [unwired: 1 out]
      n278 = dll-call lib="PTH2uabs CUsersJaehongDesktop연구_programNeuroSky_최종본NeuroSky_Dll_CallDebugNeuroSky_Dll_Call.dll" fn="FreeConnection"() -> ()  [unwired: 4 in, 2 out]
      n279 = global write "Control_Panel_정리.vi" "Acquisition Mode"(FALSE ("Device Control Enabled")) -> ()
      n280 = global write "Control_Panel_정리.vi" "Communication Stopped"(TRUE ("Device Control Enabled")) -> ()
      n281 = Build Path(base path=w750, name or relative path="Brain.txt") -> (appended path=w789:path)
      n282 = Build Path(base path=w750, name or relative path="selectedtarget.txt") -> (appended path=w781:path)
      n283 = Build Path(base path=w750, name or relative path="mius_flash_order.txt") -> (appended path=w786:path)
      n284 = Build Path(base path=w750, name or relative path="Target_order.txt") -> (appended path=w776:path)
      n285 = Build Path(base path=w750, name or relative path="Accuracy.txt") -> (appended path=w779:path)
      n286 = Build Path(base path=w750, name or relative path="ERP_발생_total.txt") -> (appended path=w769:path)
      n287 = Build Path(base path=w750, name or relative path="ERP_all_icon.txt") -> (appended path=w765:path)
      n288 = Build Path(base path=w750, name or relative path="ERP_total.txt") -> (appended path=w753:path)
      n289 = Build Path(base path=w750, name or relative path="SWLDA_hyperplane_value.txt") -> (appended path=w761:path)
      n290 = Build Path(base path=w750, name or relative path="decision_value.txt") -> (appended path=w758:path)
      n291 = call-poly <vilib>:"Write To Spreadsheet File.vi"("format (%.3f)"="%.6f", "2D data"=w745, "file path (dialog if empty)"=w789) -> ()  [unwired: 5 in, 1 out]
      n292 = call-poly <vilib>:"Write To Spreadsheet File.vi"("1D data"=w780, "file path (dialog if empty)"=w781) -> ()  [unwired: 6 in, 1 out]
      n293 = call-poly <vilib>:"Write To Spreadsheet File.vi"("transpose? (no:F)"=TRUE, "2D data"=w784, "file path (dialog if empty)"=w786) -> ()  [unwired: 5 in, 1 out]
      n294 = call-poly <vilib>:"Write To Spreadsheet File.vi"("transpose? (no:F)"=TRUE, "1D data"=w773, "file path (dialog if empty)"=w776) -> ()  [unwired: 5 in, 1 out]
      n295 = call-poly <vilib>:"Write To Spreadsheet File.vi"("1D data"=w777, "file path (dialog if empty)"=w779) -> ()  [unwired: 6 in, 1 out]
      n296 = call-poly <vilib>:"Write To Spreadsheet File.vi"("transpose? (no:F)"=TRUE, "1D data"=w767, "file path (dialog if empty)"=w769) -> ()  [unwired: 5 in, 1 out]
      n297 = call-poly <vilib>:"Write To Spreadsheet File.vi"("transpose? (no:F)"=TRUE, "format (%.3f)"="%.6f", "2D data"=w762, "file path (dialog if empty)"=w765) -> ()  [unwired: 4 in, 1 out]
      n298 = call-poly <vilib>:"Write To Spreadsheet File.vi"("transpose? (no:F)"=TRUE, "format (%.3f)"="%.6f", "2D data"=w751, "file path (dialog if empty)"=w753) -> ()  [unwired: 4 in, 1 out]
      n299 = call-poly <vilib>:"Write To Spreadsheet File.vi"("format (%.3f)"="%.6f", "1D data"=w759, "file path (dialog if empty)"=w761) -> ()  [unwired: 5 in, 1 out]
      n300 = call-poly <vilib>:"Write To Spreadsheet File.vi"("format (%.3f)"="%.6f", "1D data"=w756, "file path (dialog if empty)"=w758) -> ()  [unwired: 5 in, 1 out]
    }
    frame #4 {
      n301 = global write "Control_Panel_정리.vi" "Communication Stopped"(FALSE ("Device Control Enabled")) -> ()
    }
  }
